vi "Calculate Error Bar Vertices.vi"(4 "Error Mode":T1(ring), 6 "Marker Size":dbl, 8 "error in (no error)":errorcluster, 9 "Base Cluster":T3, 10 "Vertex Cluster":T2, 11 "Plot Area Ref":refnum<vi>) -> (0 "error out":errorcluster, 1 "Error Bar Vertex":cluster{"X":i16, "Y":i16}[][](array[cluster]), 3 "Dup Plot Area Ref":refnum<vi>)   [LabVIEW 2020, in "2D Error Bar.lvclass"]
uses:
  <vilib>/Math Plots/2D Math Plots/2D Error Bar/2D Error Bar/2D Error Bar.lvclass
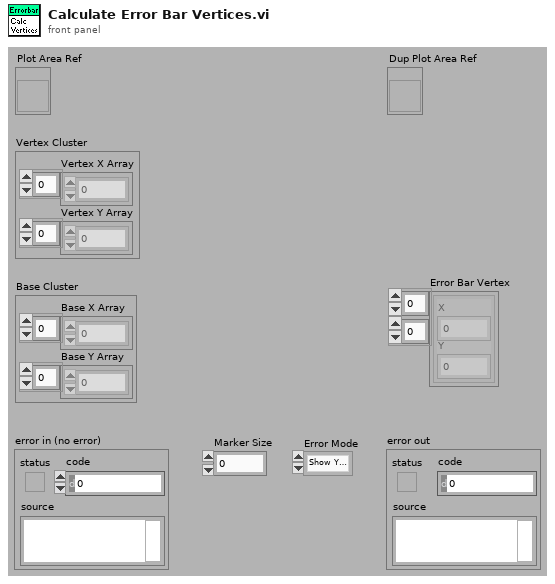
[diagram p1: front panel]
types:
  T1 = enum16{"Show Y Error", "Show X Error", "Show Both Error"}
  T2 = cluster{"Vertex X Array":dbl[], "Vertex Y Array":dbl[]}
  T3 = cluster{"Base X Array":dbl[], "Base Y Array":dbl[]}
  T4 = typedef "LVRectTypeDef.ctl" = cluster{"left":i16, "top":i16, "right":i16, "bottom":i16}
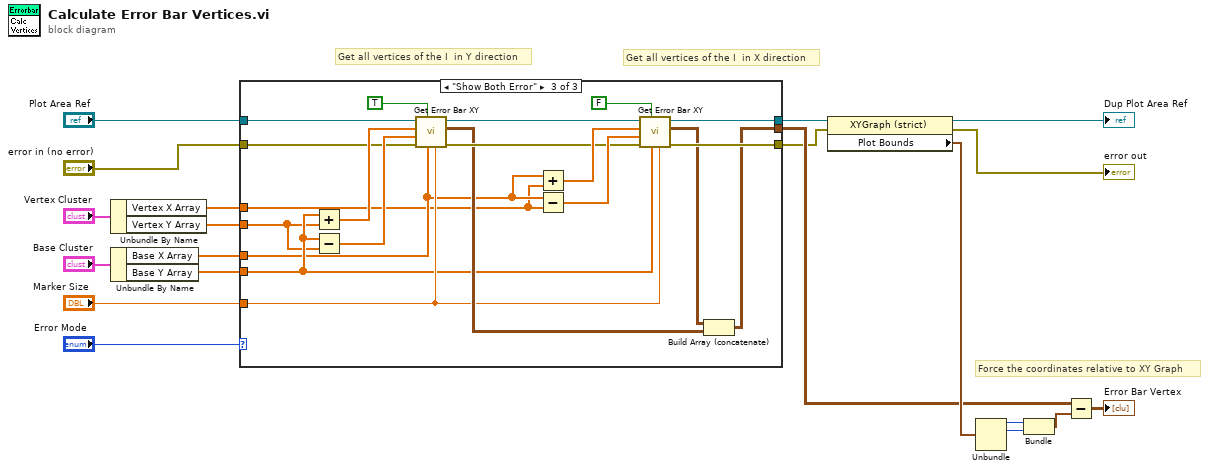
[diagram p0: block diagram]
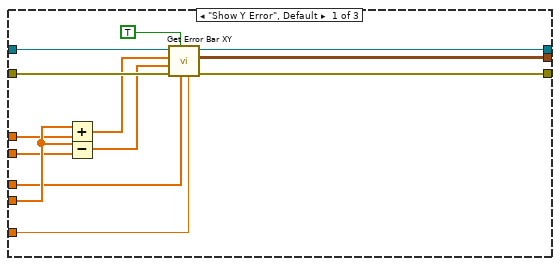
[diagram p2: hidden frame]
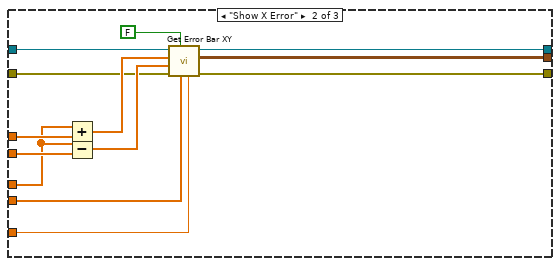
[diagram p3: hidden frame]
diagram:
  # "Get all vertices of the I  in X direction"
  # "Get all vertices of the I  in Y direction"
  # "Force the coordinates relative to XY Graph"
  n1 = Unbundle By Name("Vertex Cluster") -> ("Vertex X Array"=w5:dbl[], "Vertex Y Array"=w4:dbl[])
  n2 = Unbundle By Name("Base Cluster") -> ("Base X Array"=w2:dbl[], "Base Y Array"=w1:dbl[])
  n3 = case shown="\"Show Both Error\"" "Error Mode" {
    tunnel: w2 -> [w23 w36 w48]
    tunnel: "Marker Size" -> [w22 w34 w51]
    tunnel: [w28 w40 w52] -> w8
    tunnel: w1 -> [w33 w35 w50]
    tunnel: w5 -> [w32 w38 w47]
    tunnel: w4 -> [w31 w37 w49]
    tunnel: "Plot Area Ref" -> [w30 w43 w60]
    tunnel: "error in (no error)" -> [w26 w42 w59]
    tunnel: [w29 w41 w56] -> w7
    tunnel: [w27 w39 w55] -> w6
    frame "Show Y Error", Default {
      n4 = Add(x=w33, y=w32) -> (x+y=w25:dbl[])
      n5 = Subtract(x=w33, y=w31) -> (x-y=w24:dbl[])
      n6 = call <vilib>:"Get Error Bar XY.vi"("Marker Size"=w22, "Base"=w23, "Error Y?"=TRUE, "error in (no error)"=w26, "Min"=w24, "Max"=w25, "Plot Area Ref"=w30) -> ("error out"=w27:errorcluster, "Error Bar XY"=w28:cluster{"X":i16, "X":i16}[][], "Dup Plot Area Ref"=w29:refnum<vi>)  [unwired: 2 out]
    }
    frame "Show X Error" {
      n7 = Add(x=w36, y=w38) -> (x+y=w46:dbl[])
      n8 = Subtract(x=w36, y=w37) -> (x-y=w45:dbl[])
      n9 = call <vilib>:"Get Error Bar XY.vi"("Marker Size"=w34, "Base"=w35, "Error Y?"=FALSE, "error in (no error)"=w42, "Min"=w45, "Max"=w46, "Plot Area Ref"=w43) -> ("error out"=w39:errorcluster, "Error Bar XY"=w40:cluster{"X":i16, "X":i16}[][], "Dup Plot Area Ref"=w41:refnum<vi>)  [unwired: 2 out]
    }
    frame "Show Both Error" {
      n10 = Add(x=w50, y=w49) -> (x+y=w66:dbl[])
      n11 = Subtract(x=w50, y=w49) -> (x-y=w65:dbl[])
      n12 = call <vilib>:"Get Error Bar XY.vi"("Marker Size"=w51, "Base"=w48, "Error Y?"=TRUE, "error in (no error)"=w59, "Min"=w65, "Max"=w66, "Plot Area Ref"=w60) -> ("error out"=w57:errorcluster, "Error Bar XY"=w53:cluster{"X":i16, "X":i16}[][], "Dup Plot Area Ref"=w58:refnum<vi>)  [unwired: 2 out]
      n13 = Add(x=w48, y=w47) -> (x+y=w63:dbl[])
      n14 = Subtract(x=w48, y=w47) -> (x-y=w62:dbl[])
      n15 = call <vilib>:"Get Error Bar XY.vi"("Marker Size"=w51, "Base"=w50, "Error Y?"=FALSE, "error in (no error)"=w57, "Min"=w62, "Max"=w63, "Plot Area Ref"=w58) -> ("error out"=w55:errorcluster, "Error Bar XY"=w54:cluster{"X":i16, "X":i16}[][], "Dup Plot Area Ref"=w56:refnum<vi>)  [unwired: 2 out]
      n16 = Build Array (concatenate)(w54, w53) -> (w52:cluster{"X":i16, "X":i16}[][])
    }
  }
  n17 = property class="XYGraph (strict)"(reference=w7, error in=w6) -> (reference out=→"Dup Plot Area Ref":refnum<vi>, error out=→"error out":errorcluster, "Plot Bounds"=w17:T4)
  n18 = Unbundle(w17) -> ("left"=w15:i16, "top"=w16:i16)  [unwired: 2 out]
  n19 = Bundle("left"=w15, "top"=w16) -> (w10:cluster{"left":i16, "top":i16})  [unwired: 1 out]
  n20 = Subtract(x=w8, y=w10) -> (x-y=→"Error Bar Vertex":cluster{i16, i16}[][])
